vi "Configure Channel.vi"(0 "VISA resource name":refnum<visa-resource-name>, 1 "Vertical Scale (5.0 V)":dbl=5.0, 2 "Enable Channel (T: Enable)":bool=TRUE, 3 "Impedance (0: 1 MOhm)":i32(ring) items=["1 MOhm", "50 Ohm"], 5 "Channel Name (0: Channel 1)":i32(ring) items=["Channel 1", "Channel 2", "Channel 3", "Channel 4"], 7 "Coupling (1: DC)":i32(ring)=1 items=["AC", "DC"], 9 "Vertical Range (40.0 V)":dbl=40.0, 11 "error in (no error)":errorcluster, 12 "Vertical Offset (0.0)":dbl, 13 "Probe Attenuation (1.0)":dbl=1.0, 14 "Vertical Setting (1: Vertical Range)":i32(ring)=1 items=["Vertical Scale", "Vertical Range"]) -> (4 "VISA resource name out":refnum<visa-resource-name>, 15 "error out":errorcluster)   [LabVIEW 2017, in "Agilent 2000 3000 X-Series.lvlib"]
doc: "Configures the common properties of the vertical subsystem of the oscilloscope for the specified channel. Call this VI for each channel you want to enable to acquire waveforms.\n\n<B>Note(s):</B>\nThe channel settings will not be applied if the channel is not enabled."
uses:
  Agilent 2000 3000 X-Series.lvlib
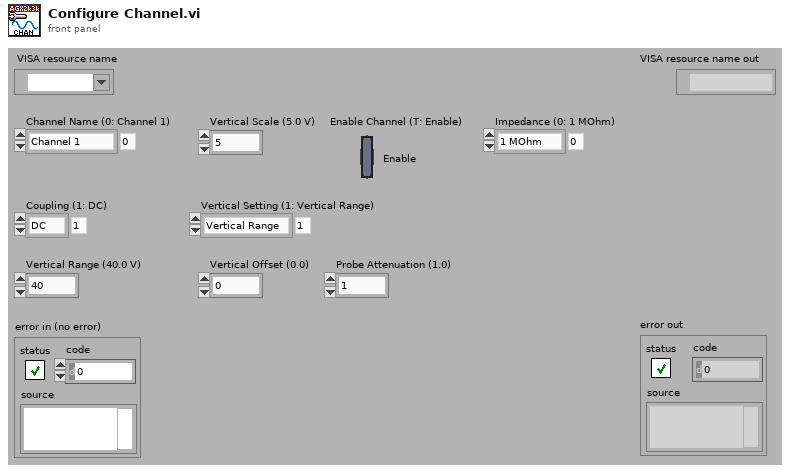
[diagram p1: front panel]
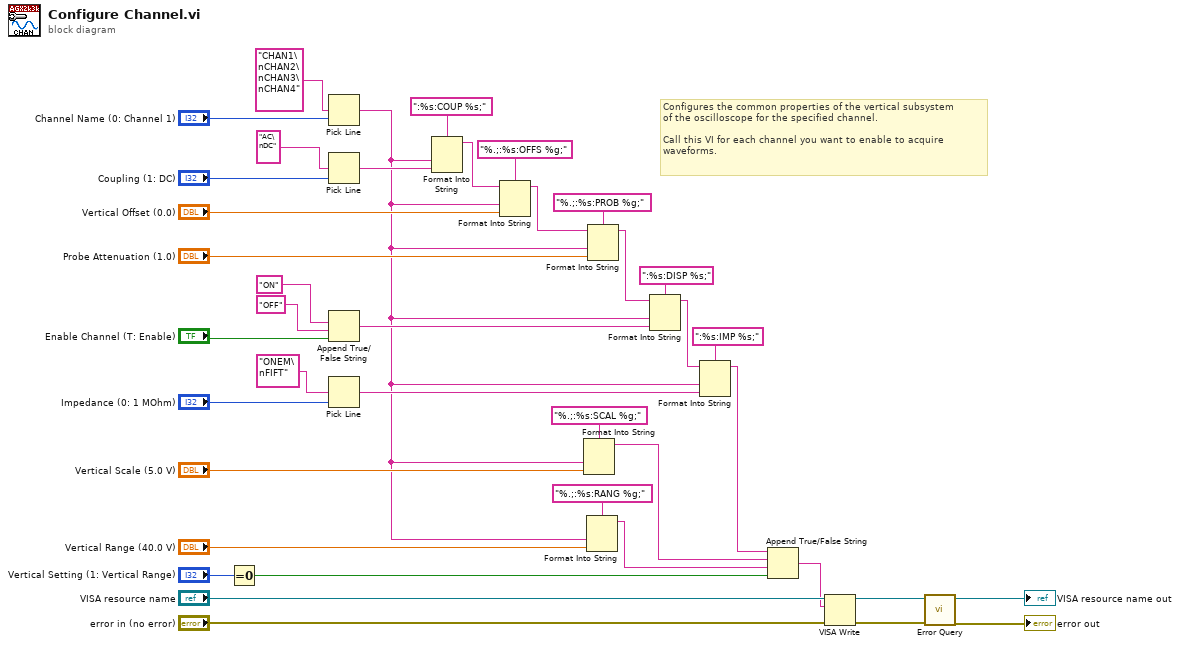
[diagram p0: block diagram]
diagram:
  # "Configures the common properties of the vertical subsystem \nof the oscilloscope for the specified channel. \n \nCall this VI for each channel you want to enable to acquire \nwaveforms."
  n1 = Equal To 0?(x="Vertical Setting (1: Vertical Range)") -> (x = 0?=w2:bool)
  n2 = Pick Line(multi-line string="CHAN1\nCHAN2\nCHAN3\nCHAN4", line index="Channel Name (0: Channel 1)") -> (output string=w6:string)  [unwired: 1 out]
  n3 = Pick Line(multi-line string="AC\nDC", line index="Coupling (1: DC)") -> (output string=w37:string)  [unwired: 1 out]
  n4 = Append True/False String(1:"Enable Channel (T: Enable)", 2:"OFF", 3:"ON") -> (0:w25:string)  [unwired: 1 out]
  n5 = Pick Line(multi-line string="ONEM\nFIFT", line index="Impedance (0: 1 MOhm)") -> (output string=w20:string)  [unwired: 1 out]
  n6 = Format Into String(format string=":%s:COUP %s;", w6, w37) -> (resulting string=w36:string)  [unwired: 2 in, 1 out]
  n7 = Format Into String(format string="%.;:%s:OFFS %g;", initial string=w36, w6, "Vertical Offset (0.0)") -> (resulting string=w9:string)  [unwired: 1 in, 1 out]
  n8 = Format Into String(format string="%.;:%s:SCAL %g;", w6, "Vertical Scale (5.0 V)") -> (resulting string=w4:string)  [unwired: 2 in, 1 out]
  n9 = Format Into String(format string="%.;:%s:RANG %g;", w6, "Vertical Range (40.0 V)") -> (resulting string=w3:string)  [unwired: 2 in, 1 out]
  n10 = Format Into String(format string="%.;:%s:PROB %g;", initial string=w9, w6, "Probe Attenuation (1.0)") -> (resulting string=w27:string)  [unwired: 1 in, 1 out]
  n11 = Format Into String(format string=":%s:DISP %s;", initial string=w27, w6, w25) -> (resulting string=w22:string)  [unwired: 1 in, 1 out]
  n12 = Format Into String(format string=":%s:IMP %s;", initial string=w22, w6, w20) -> (resulting string=w5:string)  [unwired: 1 in, 1 out]
  n13 = Append True/False String(1:w2, 2:w3, 3:w4, 4:w5) -> (0:w1:string)
  n14 = VISA Write(VISA resource name="VISA resource name", write buffer=w1, error in (no error)="error in (no error)") -> (VISA resource name out=w15:refnum<visa-resource-name>, error out=w14:errorcluster)  [unwired: 1 out]
  n15 = call "Error Query.vi"("error in (no error)"=w14, "VISA resource name"=w15) -> ("error out"=→"error out":errorcluster, "VISA resource name out"=→"VISA resource name out":refnum<visa-resource-name>)  [unwired: 8 out]
